vi "Command Page.vi"(8 "error in (no error)":errorcluster, 11 "Node Ptr":T1 format="%.0x") -> (0 "error out":errorcluster)   [LabVIEW 2027, in "Embedded Data Logger System Explorer.lvlib"]
uses:
  Embedded Data Logger System Explorer.lvlib
  <vilib>/NI VeriStand/Custom Device API/Custom Device Item Ref.ctl
  <vilib>/NI VeriStand/Custom Device API/Custom Device API.lvlib
panel:
  in  "Header":cluster{"Section Name":string}={"Section Name"="Command Channel Settings"}
  out "Description":string
  in  "Name":string
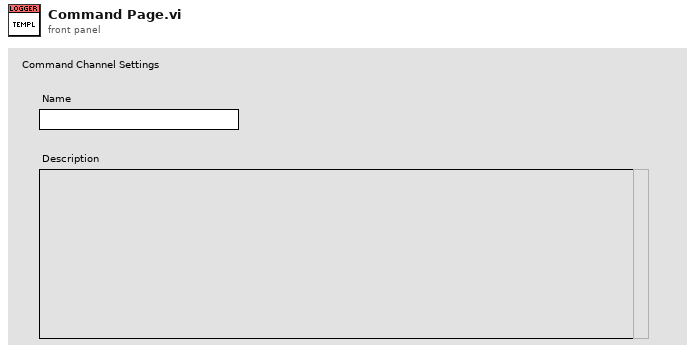
[diagram p1: front panel]
types:
  T1 = typedef "Custom Device API.lvlib/Custom Device Item Ref.ctl" = u64
  T2 = typedef "Custom Device API.lvlib/Custom Device Item Info.ctl" = cluster{"Name":string, "Is Channel":bool, "GUID":string, "Is Waveform":bool}
  T3 = typedef "Custom Device API.lvlib/Custom Device Commands.ctl" = enum16{"Default", "Item renamed", "Shutdown", "Dynamic button pressed"}
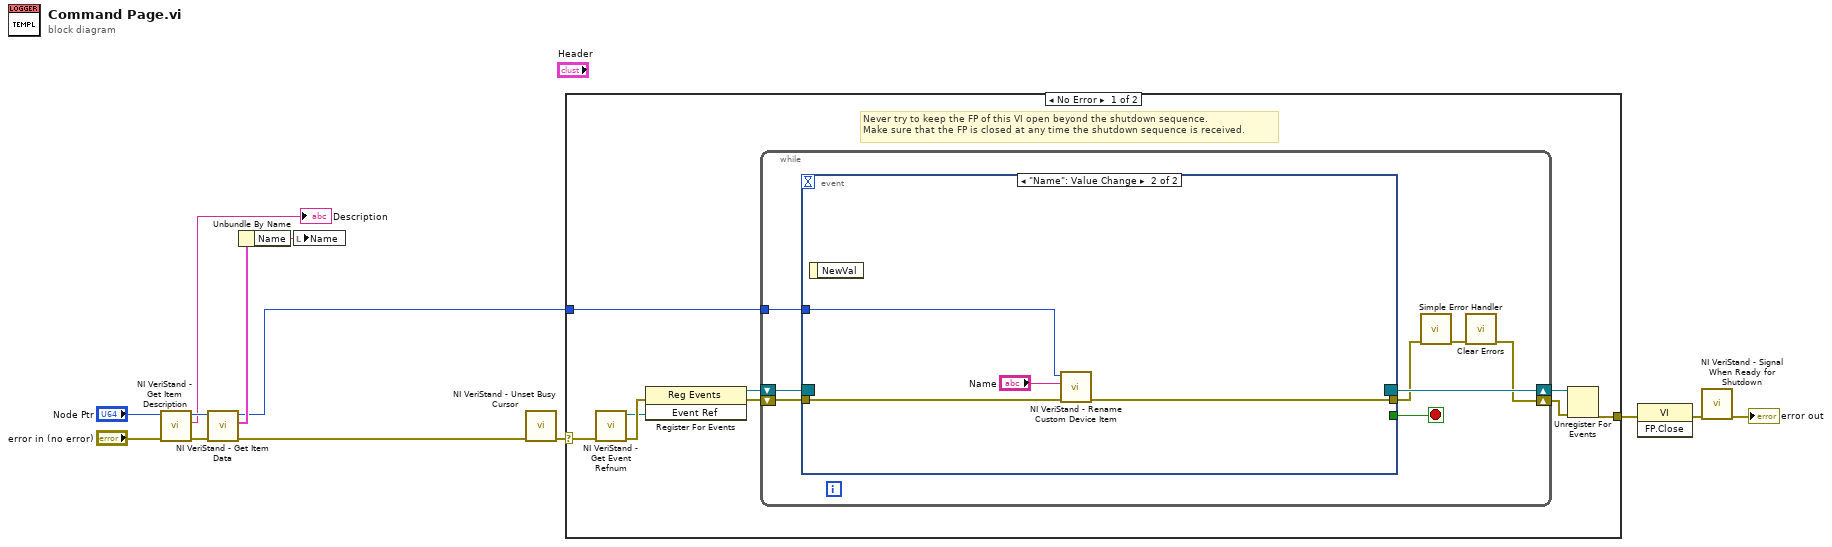
[diagram p0: block diagram]
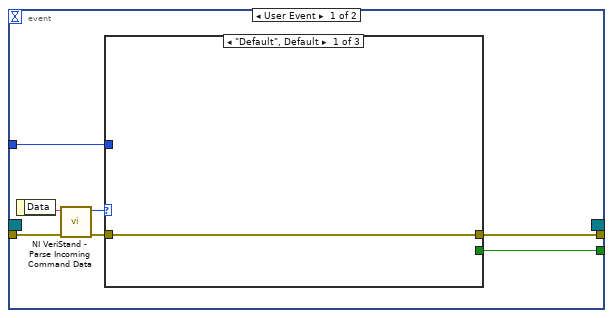
[diagram p2: hidden frame]
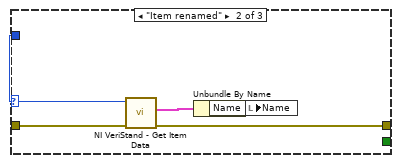
[diagram p3: hidden frame]
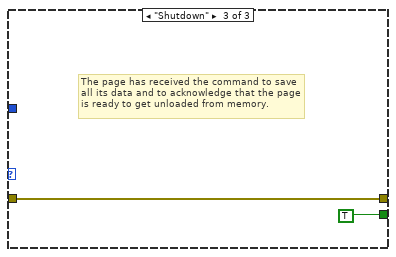
[diagram p4: hidden frame]
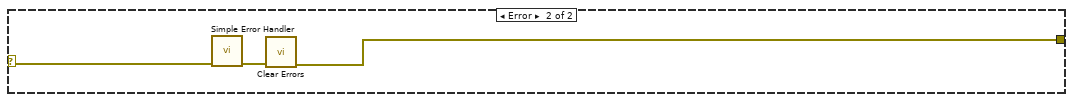
[diagram p5: hidden frame]
diagram:
  n1 = call <vilib>:"NI VeriStand - Get Item Description.vi"("error in (no error)"="error in (no error)", "Item Ref in"="Node Ptr") -> ("error out"=w6:errorcluster, "Description"=→"Description":string, "Item Ref out"=w7:T1)  [unwired: 7 out]
  n2 = call <vilib>:"NI VeriStand - Get Item Data.vi"("error in (no error)"=w6, "Item Ref in"=w7) -> ("error out"=w2:errorcluster, "Item Info"=w5:T2, "Item Ref out"=w3:T1)  [unwired: 7 out]
  n3 = Unbundle By Name(w5) -> ("Name"=w4:string)
  n4 = local write "Name"(w4) -> ()
  n5 = call <vilib>:"NI VeriStand - Unset Busy Cursor.vi"("error in (no error)"=w2) -> ("error out"=w9:errorcluster)  [unwired: 10 out]
  n6 = case shown="No Error" w9 {
    selector: w9 -> [w14 w52]
    tunnel: [w19 w50] -> w13
    tunnel: w3 -> [w15 _]
    frame No Error {
      # "Never try to keep the FP of this VI open beyond the shutdown sequence.\nMake sure that the FP is closed at any time the shutdown sequence is received."
      n7 = call <vilib>:"NI VeriStand - Get Event Refnum.vi"("error in (no error)"=w14) -> ("error out"=w22:errorcluster, "Event Ref"=w18:refnum<user-event>)  [unwired: 9 out]
      n8 = register-events(error in=w22, w18) -> (reference out=w16:refnum<event-registration>, error out=w17:errorcluster)  [unwired: 1 in]
      n9 = while {
        tunnel: w15 -> [w26]
        shift-right: [w23] -> w20
        shift-left: w17 -> [w29]
        shift-right: [w30] -> w21
        shift-left: w16 -> [w28]
        stop <- w27 stop-if-true
        n10 = event shown="[1] \"Name\": Value Change" {
          selector: w28 -> [_ _]
          dyn-events: [_ _] -> w30
          timeout: _ -> [_ _]
          tunnel: w29 -> [w37 w49]
          tunnel: [w33 _] -> w27
          tunnel: [w32 w48] -> w25
          tunnel: w26 -> [w31 w47]
          event User Event {
            n11 = event-data() -> ("Data"=w36:string)  [unwired: 1 out]
            n12 = call <vilib>:"NI VeriStand - Parse Incoming Command Data.vi"("error in (no error)"=w37, "Incoming data"=w36) -> ("error out"=w35:errorcluster, "Action"=w34:T3)  [unwired: 8 out]
            n13 = case shown="\"Default\", Default" w34 {
              tunnel: w35 -> [w38 w43 w44]
              tunnel: [_ _ TRUE] -> w33
              tunnel: [w38 w40 w44] -> w32
              tunnel: w31 -> [_ w42 _]
              frame "Default", Default {
              }
              frame "Item renamed" {
                n14 = call <vilib>:"NI VeriStand - Get Item Data.vi"("error in (no error)"=w43, "Item Ref in"=w42) -> ("error out"=w40:errorcluster, "Item Info"=w41:T2)  [unwired: 8 out]
                n15 = Unbundle By Name(w41) -> ("Name"=w39:string)
                n16 = local write "Name"(w39) -> ()
              }
              frame "Shutdown" {
                # "The page has received the command to save all its data and to acknowledge that the page is ready to get unloaded from memory."
              }
            }
          }
          event "Name": Value Change {
            n17 = event-data() -> ()  [unwired: 2 out]
            n18 = call <vilib>:"NI VeriStand - Rename Custom Device Item.vi"("error in (no error)"=w49, "New Name"="Name", "Item Ref in"=w47) -> ("error out"=w48:errorcluster)  [unwired: 1 in, 7 out]
          }
        }
        n19 = call <vilib>:"Simple Error Handler.vi"("error in (no error)"=w25) -> ("error out"=w24:errorcluster)  [unwired: 1 in, 7 out]
        n20 = call <vilib>:"Clear Errors.vi"("error in (no error)"=w24) -> ("error out"=w23:errorcluster)  [unwired: 1 in, 5 out]
      }
      n21 = Unregister For Events(event registration refnum=w21, error in=w20) -> (error out=w19:errorcluster)
    }
    frame Error {
      n22 = call <vilib>:"Simple Error Handler.vi"("error in (no error)"=w52) -> ("error out"=w51:errorcluster)  [unwired: 1 in, 7 out]
      n23 = call <vilib>:"Clear Errors.vi"("error in (no error)"=w51) -> ("error out"=w50:errorcluster)  [unwired: 1 in, 5 out]
    }
  }
  n24 = invoke class="VI" method="FP.Close"(error in=w13) -> (error out=w12:errorcluster)  [unwired: 2 in, 2 out]
  n25 = call <vilib>:"NI VeriStand - Signal When Ready for Shutdown.vi"("error in (no error)"=w12) -> ("error out"=→"error out":errorcluster)  [unwired: 10 out]
